vi "Get Last Buffer.vi"(8 "error in (no error)":errorcluster, 11 "DAQ Class in":refnum<class "DAQ Class.lvclass">) -> (0 "error out":errorcluster, 2 "Last Buffer":u16[](array[numeric]), 3 "DAQ Class out":refnum<class "DAQ Class.lvclass">)   [LabVIEW 2014, in "DAQ Class.lvclass"]
uses:
  DAQ Class.lvclass
  DAQ Class.lvclass/DAQ Class.ctl
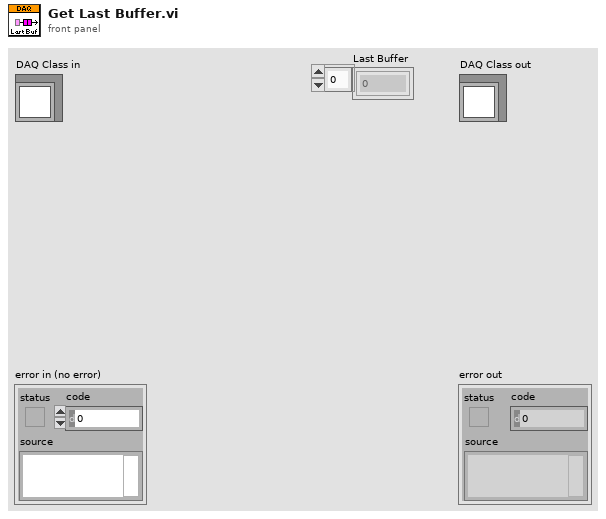
[diagram p1: front panel]
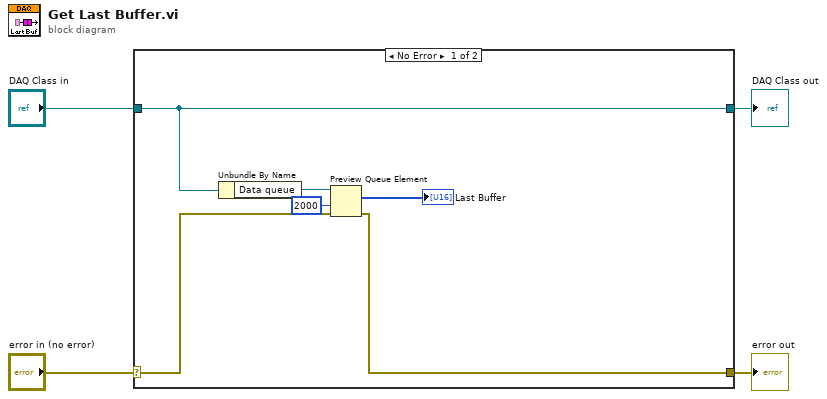
[diagram p0: block diagram]
diagram:
  n1 = case shown="No Error" "error in (no error)" {
    selector: "error in (no error)" -> [w9 w12]
    tunnel: [w8 w12] -> w3
    tunnel: [w6 w11] -> w1
    tunnel: "DAQ Class in" -> [w6 w11]
    frame No Error {
      n2 = Unbundle By Name(w6) -> ("Data queue"=w10:refnum<queue>)
      n3 = Preview Queue Element(queue=w10, timeout in ms (-1)=2000, error in (no error)=w9) -> (element=→"Last Buffer":u16[], error out=w8:errorcluster)  [unwired: 2 out]
    }
    frame Error {
    }
  }
  "error out" <- w3
  "DAQ Class out" <- w1
